vi "glsl_set_texture_string.vi"(5 "Uniform Value":dbl[][][](array[numeric]), 6 "uniform index":i32, 7 "initial string":string) -> (3 "Uniform-setting string":string)   [LabVIEW 2010]
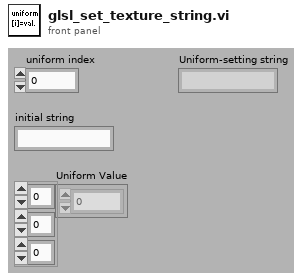
[diagram p1: front panel]
types:
  T1 = enum16{"big-endian, network order", "native, host order", "little-endian"}
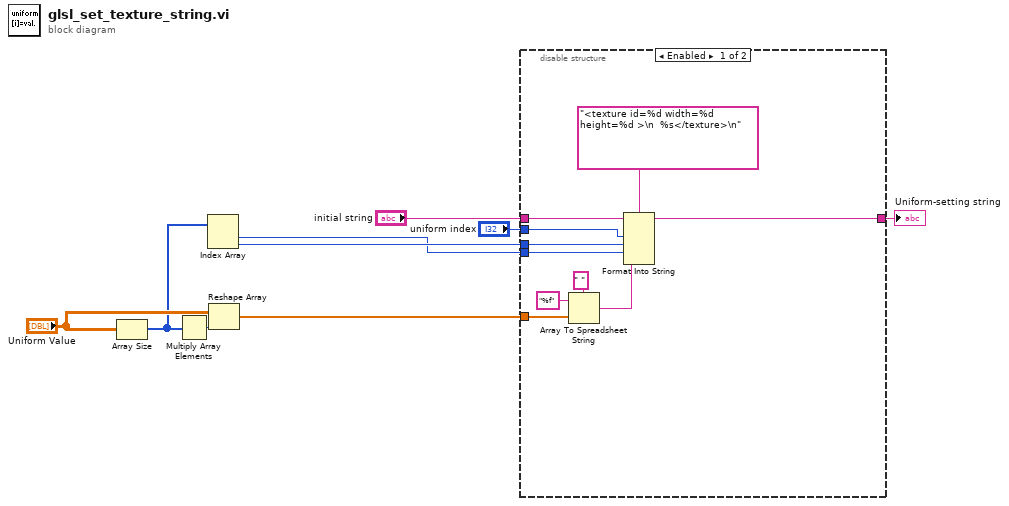
[diagram p0: block diagram]
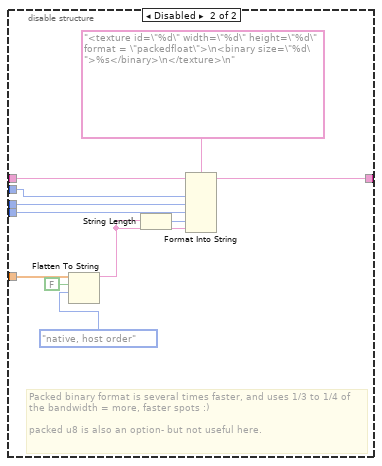
[diagram p2: hidden frame]
diagram:
  n1 = Array Size(array="Uniform Value") -> (size(s)=w5:i32[])
  n2 = Multiply Array Elements(1:w5) -> (0:w7:i32)
  n3 = Index Array(array=w5) -> (element #1=w2:i32, element #2=w3:i32)  [unwired: 2 in]
  n4 = Reshape Array("Uniform Value", w7) -> (w1:dbl[])
  n5 = disable-structure shown="Enabled" {
    disable-tunnel: "initial string" -> [w19 w30]
    disable-tunnel: [w17 w28] -> w8
    disable-tunnel: "uniform index" -> [w16 w27]
    disable-tunnel: w3 -> [w15 w26]
    disable-tunnel: w2 -> [w14 w25]
    disable-tunnel: w1 -> [w10 w23]
    frame Enabled {
      n6 = Array To Spreadsheet String(delimiter (Tab)=" ", array=w10, 3:"%f" ("format string")) -> (spreadsheet string=w11:string)
      n7 = Format Into String(format string="<texture id=%d width=%d height=%d >\n  %s</texture>\n", initial string=w19, w16, w15, w14, w11) -> (resulting string=w17:string)  [unwired: 1 in, 1 out]
    }
    frame Disabled {
      # "Packed binary format is several times faster, and uses 1/3 to 1/4 of the bandwidth = more, faster spots :)\n\npacked u8 is also an option- but not useful here."
      n8 = Flatten To String(anything=w23, prepend array or string size? (T)=FALSE, byte order (0:big-endian, network order)=T1."native, host order") -> (data string=w20:string)  [unwired: 1 in, 2 out]
      n9 = String Length(string=w20) -> (length=w21:i32)
      n10 = Format Into String(format string="<texture id=\"%d\" width=\"%d\" height=\"%d\" format = \"packedfloat\">\n<binary size=\"%d\">%s</binary>\n</texture>\n" ("data in"), initial string=w30, w27, w26, w25, w21, w20) -> (resulting string=w28:string)  [unwired: 1 in, 1 out]
    }
  }
  "Uniform-setting string" <- w8
